vi "Configure Pulse Sweep.vi"(0 "VISA resource name":refnum<visa-resource-name>, 1 "Buffer Name":string="defbuffer1", 5 "Function (0:Voltage)":u16(ring) items=["Voltage", "Current"], 7 "Sweep Parameters":T1={"Bias Level (0)"=0.0, "Start (0)"=0.0, "Stop (0)"=0.0, "Sweep Type (0:Linear)"=0, "Bias Limit (.1)"=0.1, "Points (2)"=2} {"Sweep Type (0:Linear)" items=["Linear", "Log"]}, 9 "Pulse Parameters":T2={"Pulse Off Time (0.01)"=0.01, "Pulse Width (.05)"=0.05, "Delay (0)"=0.0, "Pulse Limit (.1)"=0.1}, 11 "error in (no error)":errorcluster, 12 "Enable Measure (T: Enable)":bool=TRUE) -> (4 "VISA resource name out":refnum<visa-resource-name>, 15 "error out":errorcluster)   [LabVIEW 2020, in "Keithley 2450.lvlib"]
doc: "Sets up a linear or log based pulse sweep for a fixed number of pulse points.\n\n<B>This function is only compatible with the 2461.</B>"
uses:
  Keithley 2450.lvlib
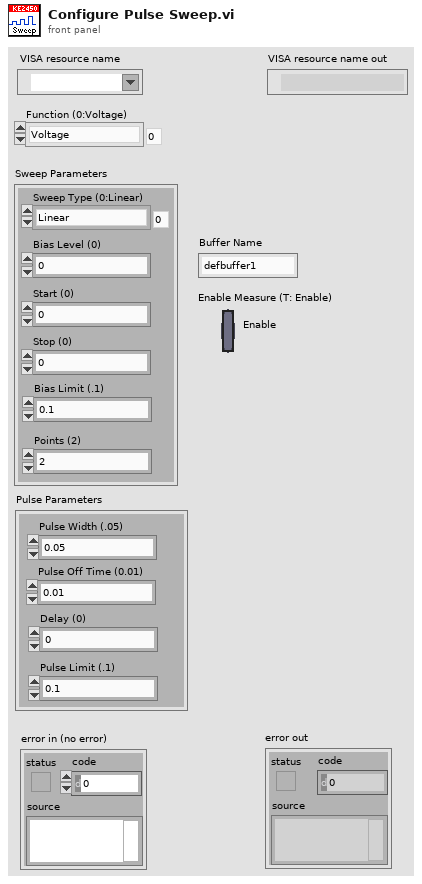
[diagram p1: front panel]
types:
  T1 = cluster{"Bias Level (0)":dbl, "Start (0)":dbl, "Stop (0)":dbl, "Sweep Type (0:Linear)":u16, "Bias Limit (.1)":dbl, "Points (2)":u16}
  T2 = cluster{"Pulse Off Time (0.01)":dbl, "Pulse Width (.05)":dbl, "Delay (0)":dbl, "Pulse Limit (.1)":dbl}
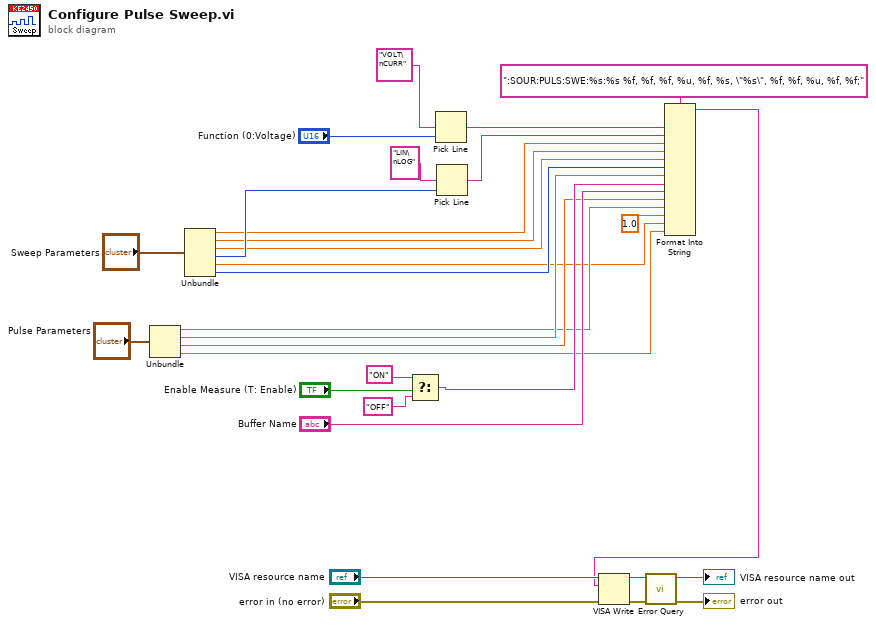
[diagram p0: block diagram]
diagram:
  n1 = Unbundle("Pulse Parameters") -> ("Pulse Off Time (0.01)"=w3:dbl, "Pulse Width (.05)"=w5:dbl, "Delay (0)"=w4:dbl, "Pulse Limit (.1)"=w1:dbl)
  n2 = Unbundle("Sweep Parameters") -> ("Bias Level (0)"=w10:dbl, "Start (0)"=w9:dbl, "Stop (0)"=w8:dbl, "Sweep Type (0:Linear)"=w11:u16, "Bias Limit (.1)"=w2:dbl, "Points (2)"=w7:u16)
  n3 = Select(t="ON", s="Enable Measure (T: Enable)", f="OFF") -> (s? t:f=w15:string)
  n4 = Pick Line(multi-line string="VOLT\nCURR", line index="Function (0:Voltage)") -> (output string=w21:string)  [unwired: 1 in]
  n5 = Pick Line(multi-line string="LIN\nLOG", line index=w11) -> (output string=w16:string)  [unwired: 1 in]
  n6 = Format Into String(format string=":SOUR:PULS:SWE:%s:%s %f, %f, %f, %u, %f, %s, \"%s\", %f, %f, %u, %f, %f;" ("multi-line string"), w21, w16, w10, w9, w8, w7, w5, w15, "Buffer Name", w4, w3, 1.0 ("input 12"), w2, w1) -> (resulting string=w23:string)  [unwired: 2 in, 1 out]
  n7 = VISA Write(VISA resource name="VISA resource name", write buffer=w23, error in (no error)="error in (no error)") -> (VISA resource name out=w27:refnum<visa-resource-name>, error out=w26:errorcluster)  [unwired: 1 out]
  n8 = call "Error Query.vi"("error in (no error)"=w26, "VISA resource name"=w27) -> ("error out"=→"error out":errorcluster, "VISA resource name out"=→"VISA resource name out":refnum<visa-resource-name>)  [unwired: 8 out]
